vi "CamStore.vi"(4 "folderpath":path, 5 "Experiment State in":T1={"error"={"status"=FALSE, "code"=0, "source"=""}, "Digitizer DAQmx Tasks"={"TaskArray"=[]}, "DAQ Settings"={"Channel Settings"=[], "Card Settings"=[]}, "Synchronization Settings"={"Synchronizer 0"="PXI1Slot2", "source terminal"="GlobalSoftwareTrigger", "Synchronizer 1"="PXI1Slot2"}, "DAQ Data"=[], "Next Shot#"="0", "System Message"="", "User Shot Notes"="", "Timing Settings"={"Timing Card Settings"=[], "Timing Channel Settings"=[[{"Delay (s)"=2.559999942779541, "Pulse width (s)"=0.009999999776482582, "Active"=TRUE, "Channel Name"="Fiber 8", "counter"="PXI1Slot8/ctr7", "FrontPanelTime"=2.559999942779541}]]}, "Timing Tasks"={"TaskArray"=[]}, "Tree"="0", "Time Card/Channels"=[2, 8], "DAQ Card/Channels"=[3, 8], "Program Version"="", "RIO Settings"={"Channel Settings"=[], "Card Settings"=[]}, "RIO References"={"Reference Array"=[]}, "RIO Data"={"RIO Deleaved Data"=[], "Raw Readout"=[]}, "RIO Card/Channels"=[3, 8], "DIO Channels"=0, "DIO Settings"={"DIO Channel Array"=[]}} {"RIO Settings"."Card Settings"."Sample Rate" format="%#_3p"; "Timing Settings"."Timing Channel Settings"."FrontPanelTime" format="%.3p"; "Timing Settings"."Timing Channel Settings"."Pulse width (s)" format="%.3p"; "Timing Settings"."Timing Channel Settings"."Delay (s)" format="%.3p"; "DAQ Settings"."Card Settings"."Global Edge Type" items=["Rising"=10280, "Falling"=10171]; "DAQ Settings"."Card Settings"."Sample Rate" format="%#_3p"}) -> (1 "cmd output":string, 2 "Experiment State out":T1={"error"={"status"=FALSE, "code"=0, "source"=""}, "Digitizer DAQmx Tasks"={"TaskArray"=[]}, "DAQ Settings"={"Channel Settings"=[], "Card Settings"=[]}, "Synchronization Settings"={"Synchronizer 0"="PXI1Slot2", "source terminal"="GlobalSoftwareTrigger", "Synchronizer 1"="PXI1Slot2"}, "DAQ Data"=[], "Next Shot#"="0", "System Message"="", "User Shot Notes"="", "Timing Settings"={"Timing Card Settings"=[], "Timing Channel Settings"=[[{"Delay (s)"=2.559999942779541, "Pulse width (s)"=0.009999999776482582, "Active"=TRUE, "Channel Name"="Fiber 8", "counter"="PXI1Slot8/ctr7", "FrontPanelTime"=2.559999942779541}]]}, "Timing Tasks"={"TaskArray"=[]}, "Tree"="0", "Time Card/Channels"=[2, 8], "DAQ Card/Channels"=[3, 8], "Program Version"="", "RIO Settings"={"Channel Settings"=[], "Card Settings"=[]}, "RIO References"={"Reference Array"=[]}, "RIO Data"={"RIO Deleaved Data"=[], "Raw Readout"=[]}, "RIO Card/Channels"=[3, 8], "DIO Channels"=0, "DIO Settings"={"DIO Channel Array"=[]}} {"RIO Settings"."Card Settings"."Sample Rate" format="%#_3p"; "Timing Settings"."Timing Channel Settings"."FrontPanelTime" format="%.3p"; "Timing Settings"."Timing Channel Settings"."Pulse width (s)" format="%.3p"; "Timing Settings"."Timing Channel Settings"."Delay (s)" format="%.3p"; "DAQ Settings"."Card Settings"."Global Edge Type" items=["Rising"=10280, "Falling"=10171]; "DAQ Settings"."Card Settings"."Sample Rate" format="%#_3p"})   [LabVIEW 2014]
uses:
  Controls/ExperimentStateCluster.ctl
  Controls/DigitizerSettingsChannelSettings.ctl
  Controls/DigitizerSettingsCardSettingsArray.ctl
  Controls/DigitizerSettingsCardSettings.ctl
  Controls/TimingSettings.ctl
  Controls/TimingCardSettings.ctl
  Controls/TimingChannelSettings.ctl
  Controls/RIOSettingsExperimentStateCluster.ctl
  Controls/RIOChannelSettingsArrayExperimentStateCluster.ctl
  Controls/RIOSettingsChannelSettings.ctl
  Controls/RIOSettingsCardSettingsArray.ctl
  Controls/RIOSettingsCardSettings.ctl
  <vilib>/userdefined/High Color/nirio_resource_hc.ctl
  Controls/RIOData.ctl
  Controls/DIOChannel.ctl
panel:
  in  "working directory":path=path "Z:/MOCHIcontrol/PythonStore/spe_file_handling"
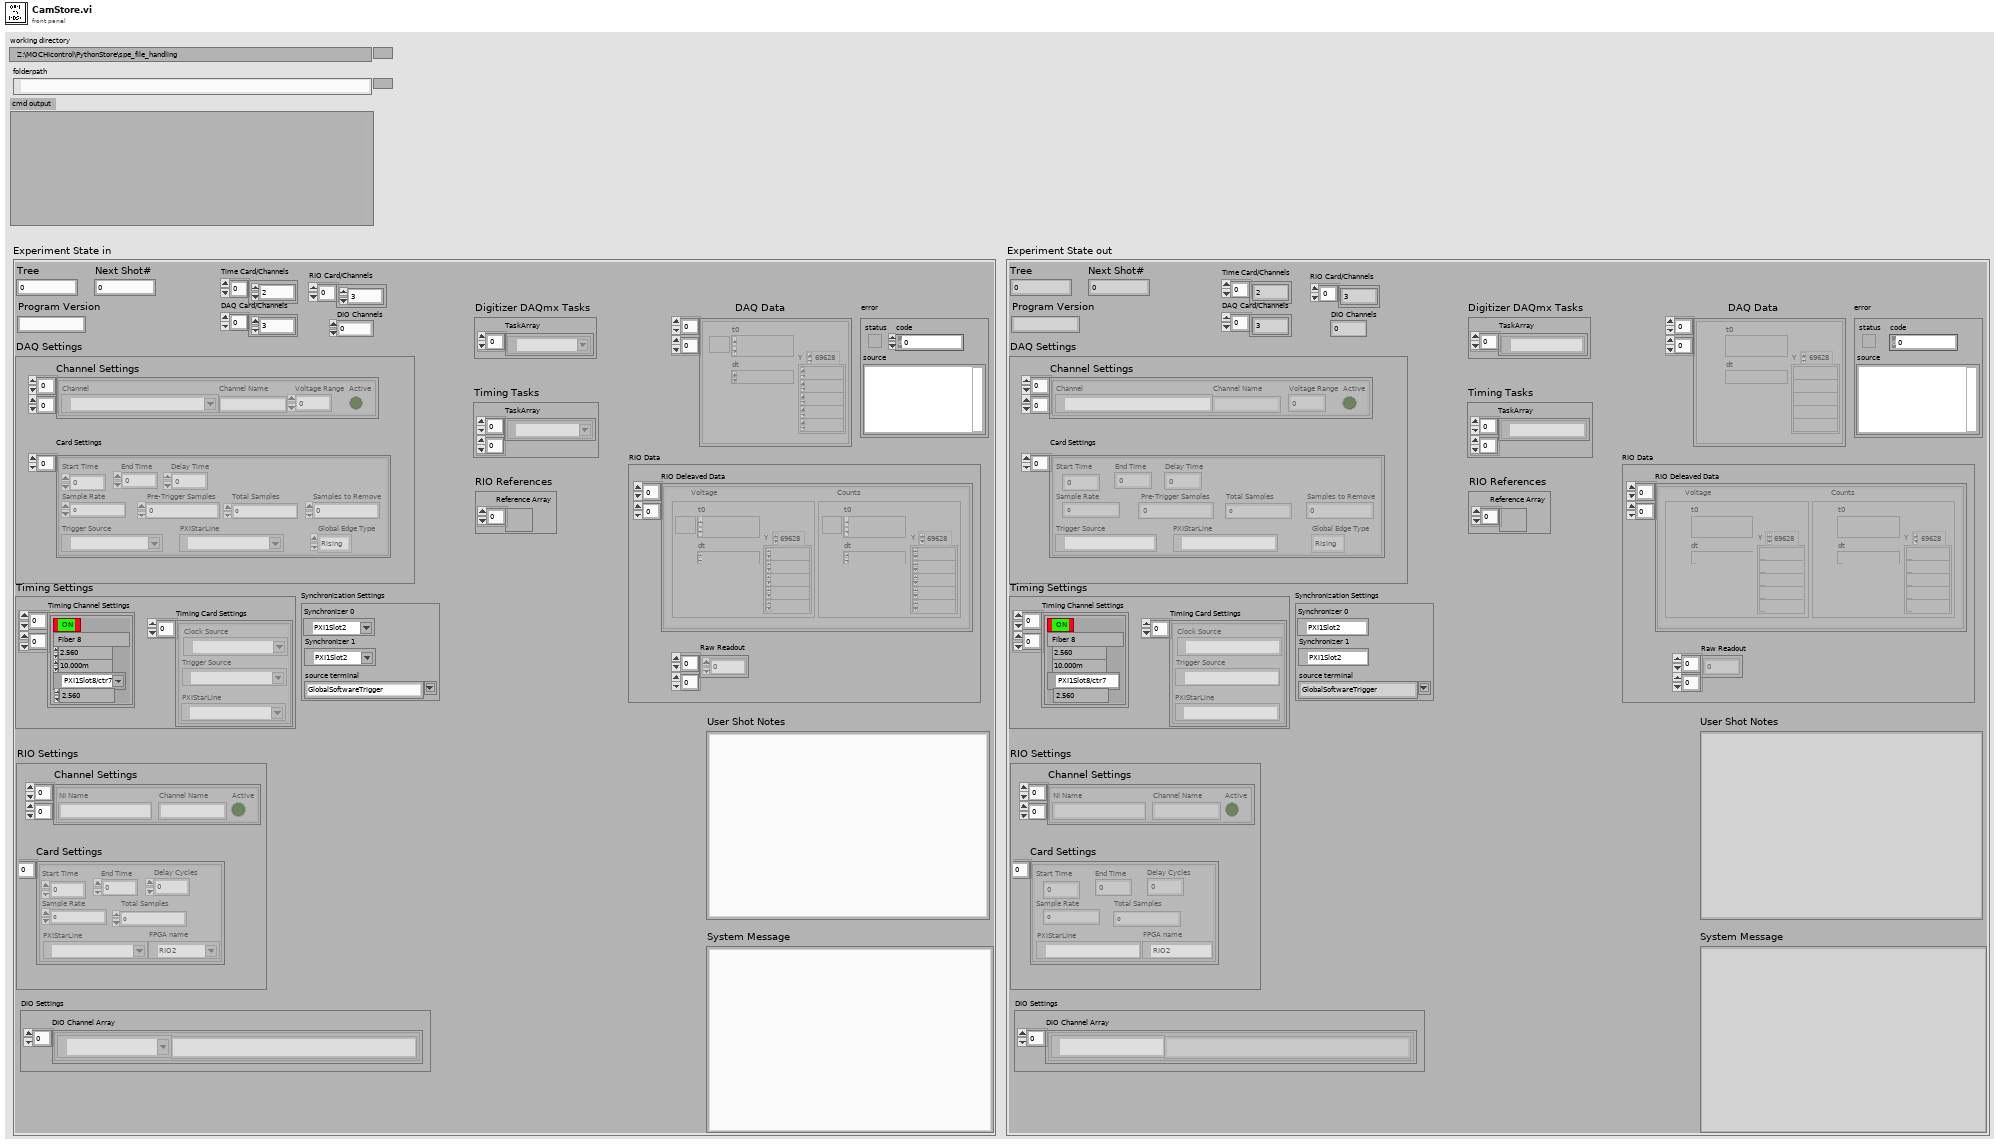
[diagram p1: front panel]
types:
  T1 = typedef "ExperimentStateCluster.ctl" = cluster{"error":errorcluster, "Digitizer DAQmx Tasks":cluster{"TaskArray":refnum<k21>[]}, "DAQ Settings":cluster{"Channel Settings":T2[][], "Card Settings":T3}, "Synchronization Settings":cluster{"Synchronizer 0":refnum<k15>, "source terminal":string, "Synchronizer 1":refnum<k15>}, "DAQ Data":waveform(dbl)[][], "Next Shot#":string, "System Message":string, "User Shot Notes":string, "Timing Settings":T5, "Timing Tasks":cluster{"TaskArray":refnum<k21>[][]}, "Tree":string, "Time Card/Channels":i32[], "DAQ Card/Channels":i32[], "Program Version":string, "RIO Settings":T8, "RIO References":cluster{"Reference Array":refnum<k20>[]}, "RIO Data":T14, "RIO Card/Channels":i32[], "DIO Channels":i32, "DIO Settings":cluster{"DIO Channel Array":T15[]}}
  T2 = typedef "DigitizerSettingsChannelSettings.ctl" = cluster{"Channel":tag, "Channel Name":string, "Voltage Range":dbl, "Active":bool}
  T3 = typedef "DigitizerSettingsCardSettingsArray.ctl" = T4[]
  T4 = typedef "DigitizerSettingsCardSettings.ctl" = cluster{"Start Time":dbl, "End Time":dbl, "Sample Rate":dbl, " Pre-Trigger Samples":u32, "Total Samples":i32, "Samples to Remove":u32, "Trigger Source":tag, "Global Edge Type":i32, "PXIStarLine":tag, "Delay Time":dbl}
  T5 = typedef "TimingSettings.ctl" = cluster{"Timing Card Settings":T6[], "Timing Channel Settings":T7[][]}
  T6 = typedef "TimingCardSettings.ctl" = cluster{"Trigger Source":tag, "Clock Source":tag, "PXIStarLine":tag}
  T7 = typedef "TimingChannelSettings.ctl" = cluster{"Delay (s)":dbl, "Pulse width (s)":dbl, "Active":bool, "Channel Name":string, "counter":tag, "FrontPanelTime":dbl}
  T8 = typedef "RIOSettingsExperimentStateCluster.ctl" = cluster{"Channel Settings":T9, "Card Settings":T11}
  T9 = typedef "RIOChannelSettingsArrayExperimentStateCluster.ctl" = T10[][]
  T10 = typedef "RIOSettingsChannelSettings.ctl" = cluster{"Channel Name":string, "Active":bool, "NI Name":string}
  T11 = typedef "RIOSettingsCardSettingsArray.ctl" = T12[]
  T12 = typedef "RIOSettingsCardSettings.ctl" = cluster{"Start Time":dbl, "End Time":dbl, "Sample Rate":dbl, "Total Samples":u64, "PXIStarLine":tag, "Delay Cycles":u64, "FPGA name":T13}
  T13 = typedef "nirio_resource_hc.ctl" = tag
  T14 = typedef "RIOData.ctl" = cluster{"RIO Deleaved Data":cluster{"Voltage":waveform(dbl), "Counts":waveform(i16)}[][], "Raw Readout":u64[][]}
  T15 = typedef "DIOChannel.ctl" = cluster{"Channel Name":string, "NI Name":tag}
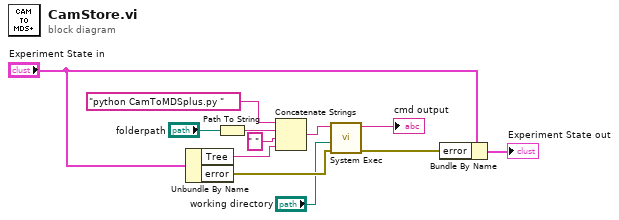
[diagram p0: block diagram]
diagram:
  n1 = Unbundle By Name("Experiment State in") -> ("Tree"=w5:string, "error"=w4:errorcluster)
  n2 = Path To String(path="folderpath") -> (string=w10:string)
  n3 = Concatenate Strings("python CamToMDSplus.py ", w10, " " ("string"), w5) -> (w9:string)
  n4 = call <vilib>:"System Exec.vi"("error in (no error)"=w4, "working directory"="working directory", "command line"=w9) -> ("error out"=w3:errorcluster, "standard output"=→"cmd output":string)  [unwired: 5 in, 2 out]
  n5 = Bundle By Name(cluster="Experiment State in", "error"=w3) -> (→"Experiment State out":T1)
